vi "Clear Error Info.vi"(11 "Base Actor in":refnum<class "Base Actor.lvclass">) -> (3 "Base Actor out":refnum<class "Base Actor.lvclass">)   [LabVIEW 2020, in "jettl.lvlib" / "Actor.lvlib" / "Base Actor.lvclass"]
uses:
  Base Actor.lvclass
  Error Info.ctl
  Actor.lvlib
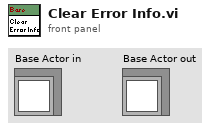
[diagram p1: front panel]
types:
  T1 = typedef "jettl.lvlib/Actor.lvlib/Error Info.ctl" = cluster{"Is Framework Error":bool, "Error":errorcluster}
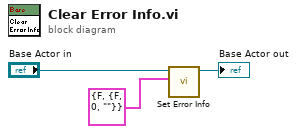
[diagram p0: block diagram]
diagram:
  n1 = call "Set Error Info.vi"("Error Info"=T1 {"Is Framework Error"=FALSE, "Error"={"status"=FALSE, "code"=0, "source"=""}}, "Base Actor in"="Base Actor in") -> ("Base Actor out"=→"Base Actor out":refnum<class "Base Actor.lvclass">)  [unwired: 9 in]
